vi "MH_DataInQueue.vi"(8 "error in (no error)":errorcluster, 10 "CountsHistos":T1, 11 "MultiharpComm in":refnum<class "MultiharpComm.lvclass">) -> (0 "error out":errorcluster, 3 "MultiharpComm out":refnum<class "MultiharpComm.lvclass">)   [LabVIEW 2023, in "MultiharpComm.lvlib" / "MultiharpComm.lvclass"]
uses:
  MultiharpComm.lvclass
  UIs/SinglePhoton_UI/Libraries/SinglePhotonInterferenceUI/CountsHistos.ctl
  typedefs/typedefs.lvlib
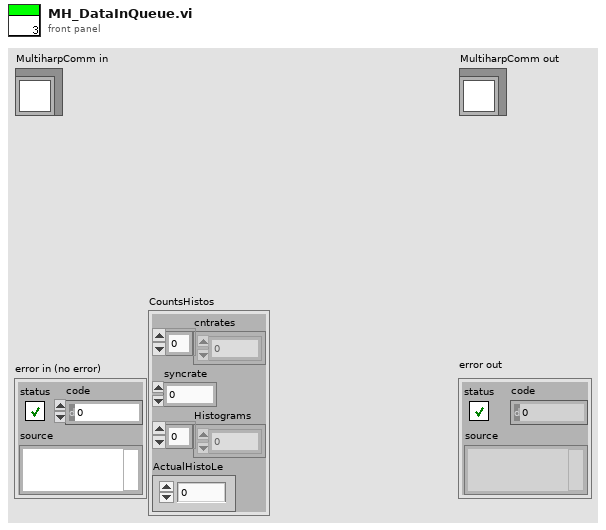
[diagram p1: front panel]
types:
  T1 = typedef "typedefs.lvlib/CountsHistos.ctl" = cluster{"cntrates":i32[], "syncrate":i32, "Histograms":u32[], "ActualHistoLe":i32}
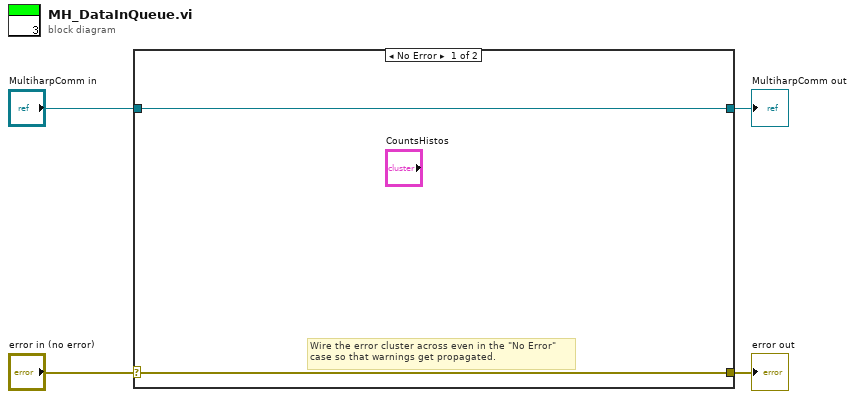
[diagram p0: block diagram]
diagram:
  n1 = case shown="No Error" "error in (no error)" {
    selector: "error in (no error)" -> [w5 w8]
    tunnel: [w5 w8] -> w3
    tunnel: [w6 w7] -> w1
    tunnel: "MultiharpComm in" -> [w6 w7]
    frame No Error {
      # "Wire the error cluster across even in the \"No Error\"\ncase so that warnings get propagated."
    }
    frame Error {
    }
  }
  "error out" <- w3
  "MultiharpComm out" <- w1
